vi "Get Hi Low Times Out Temp V.vi"(8 "error in (no error)":errorcluster, 10 "DateTimeLowOutTemp":T1, 11 "DateTimeHiOutTemp":T1) -> (0 "error out":errorcluster, 1 "function return":i16, 2 "DateTimeLowOutTemp out":T1, 3 "DateTimeHiOutTemp out":T1)   [LabVIEW 2009, in "VantagePro.lvlib"]
doc: "DllAccess short int _stdcall GetHiLowTimesOutTemp_V (DateTime* DateTimeHiOutTemp, DateTime* DateTimeLowOutTemp);"
uses:
  VantagePro.lvlib
  <userlib>/VantagePro/VantagePro.dll
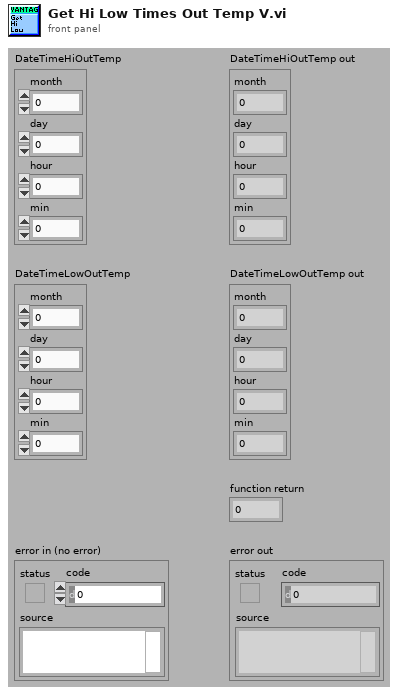
[diagram p1: front panel]
types:
  T1 = cluster{"month":i16, "day":i16, "hour":i16, "min":i16}
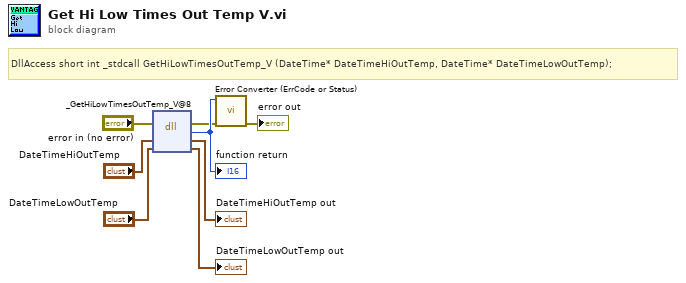
[diagram p0: block diagram]
diagram:
  # "DllAccess short int _stdcall GetHiLowTimesOutTemp_V (DateTime* DateTimeHiOutTemp, DateTime* DateTimeLowOutTemp);"
  n1 = dll-call lib="C:/Program Files/National Instruments/LabVIEW 2010/user.lib/VantagePro/VantagePro.*" fn="_GetHiLowTimesOutTemp_V@8"(error in="error in (no error)", "DateTimeHiOutTemp"="DateTimeHiOutTemp", "DateTimeLowOutTemp"="DateTimeLowOutTemp") -> (error out=w2:errorcluster, w8:i16, "DateTimeHiOutTemp"=→"DateTimeHiOutTemp out":T1, "DateTimeLowOutTemp"=→"DateTimeLowOutTemp out":T1)  [unwired: 2 in, 1 out]
  "function return" <- w8
  n2 = call "Error Converter (ErrCode or Status).vi"("error in (no error)"=w2, "error code"=w8) -> ("error out"=→"error out":errorcluster)  [unwired: 9 in]
